vi "HighestColor (2).vi"(0 "Rango":bool, 1 "ColorPrincipal":dbl, 2 "Color 1":dbl, 3 "Color 2":dbl, 4 "Color 3":dbl, 5 "Color 4":dbl) -> (14 "Resultado":bool)   [LabVIEW 2018]
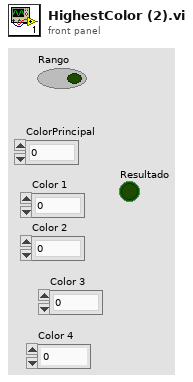
[diagram p1: front panel]
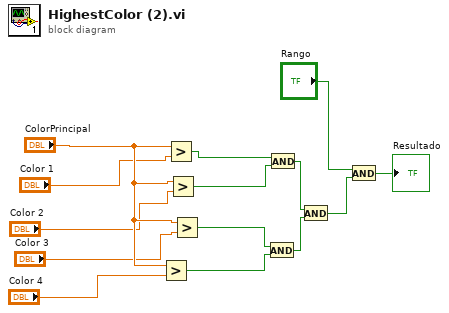
[diagram p0: block diagram]
diagram:
  n1 = Greater?(x="ColorPrincipal", y="Color 4") -> (0:w11:bool)
  n2 = Greater?(x="ColorPrincipal", y="Color 1") -> (0:w14:bool)
  n3 = Greater?(x="ColorPrincipal", y="Color 2") -> (0:w13:bool)
  n4 = Greater?(x="ColorPrincipal", y="Color 3") -> (0:w12:bool)
  n5 = And(x=w12, y=w11) -> (x .and. y?=w10:bool)
  n6 = And(x=w14, y=w13) -> (x .and. y?=w9:bool)
  n7 = And(x=w9, y=w10) -> (x .and. y?=w8:bool)
  n8 = And(x="Rango", y=w8) -> (x .and. y?=→"Resultado":bool)
